vi "Global DAQ started.vi"() -> ()   [LabVIEW 2020]
panel:
  out "DAQ Started":bool
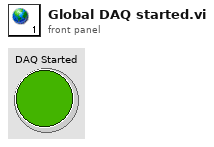
[diagram p1: front panel]
diagram:
